vi "ABB Test report .vi"() -> (0 "error out":errorcluster)   [LabVIEW 2017]
uses:
  ABB global.vi
  <vilib>/Utility/NIReport.llb/NI_report.lvclass
panel:
  in  "Sign":bool
  out "Array":cluster{"String":string, "OK Button":bool}[](array[cluster])
  out "result string":string
  in  "Save":bool
  in  "View Pages":bool
  in  "Select page":u16(ring) items=["Cover Page", "Contents", "Pass/Fail Criteria", "Rated Data", " General Information", "Measurements", "No Load Test", "Short Circuit Test", "Heat Run", "Heat Run Data", "Cooling curve", "No Load Heat Run", "Heat Run Data", "No Load Cooling curve", "Bearing Run", "Bearing Run Data", "Efficiency", "Noise", "Noise Analysis 1", "Noise Analysis 2", "Bearing Inspection", "Instruments"]
  out "Message":string="Compiling Report...."
  in  "Select None":bool
  in  "Select All":bool
  out "Pages":string[](array[string])
  in  "Include":bool[](array[boolean])
  in  "Exit":bool
  in  "Print":bool
  in  "WebBrowser":refnum<k7>(container)
  # "Test Report"
  # "Include pages"
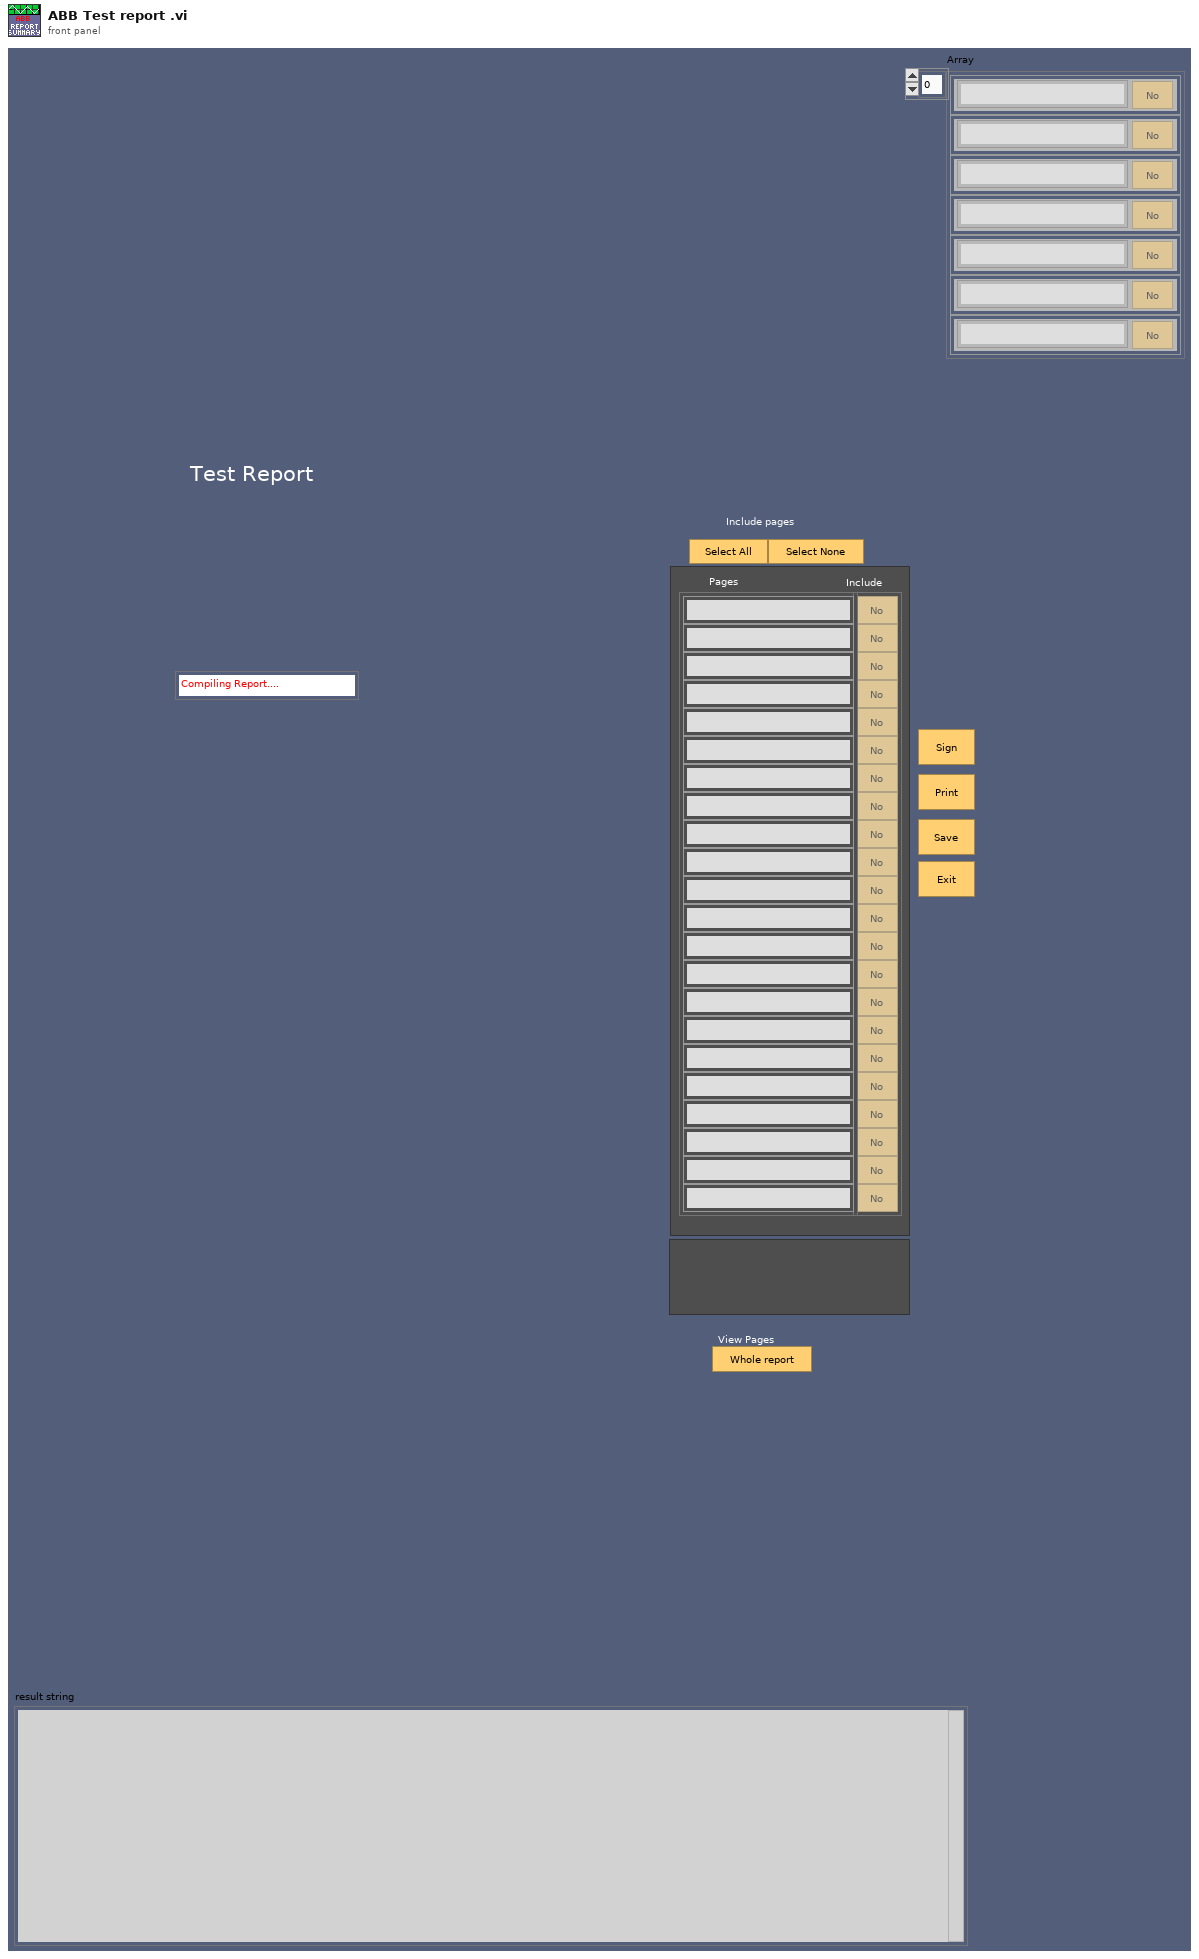
[diagram p1: front panel]
types:
  T1 = typedef "Generate Report Object Reference.ctl" = refnum<class "NI_report.lvclass">
  T2 = enum32{"existing file", "new file", "new or existing file", "existing dir", "new dir", "new or existing dir", "existing file (use LLBs)", "new file (use LLBs)", "new or existing file (use LLBs)", "new or existing file or directory (use LLBs)"}
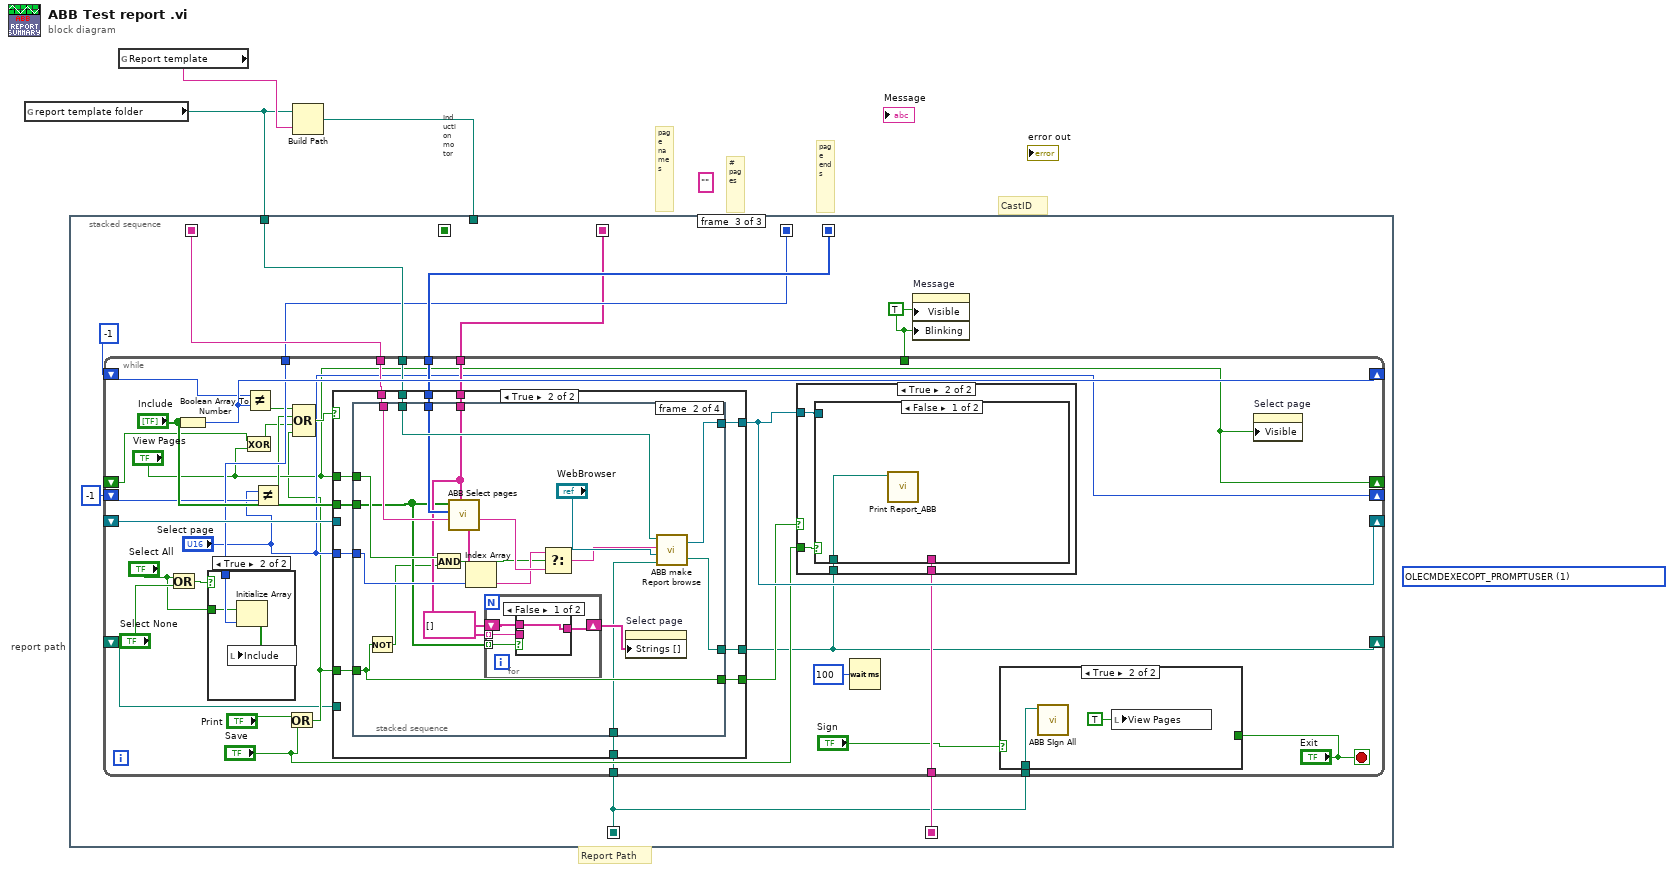
[diagram p0: block diagram]
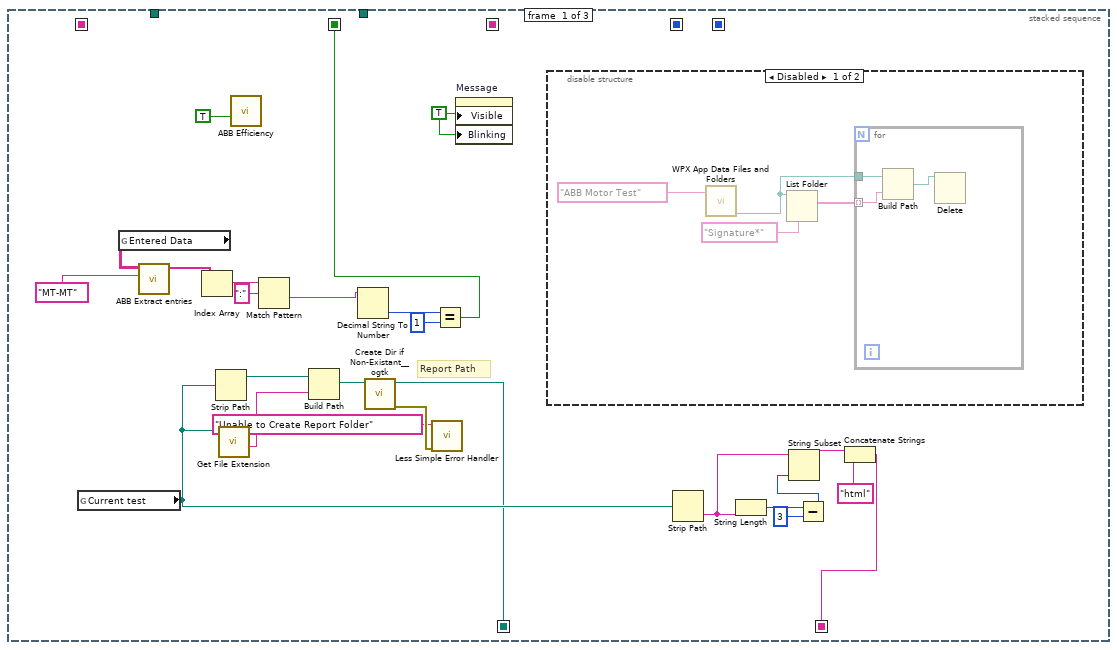
[diagram p2: hidden frame]
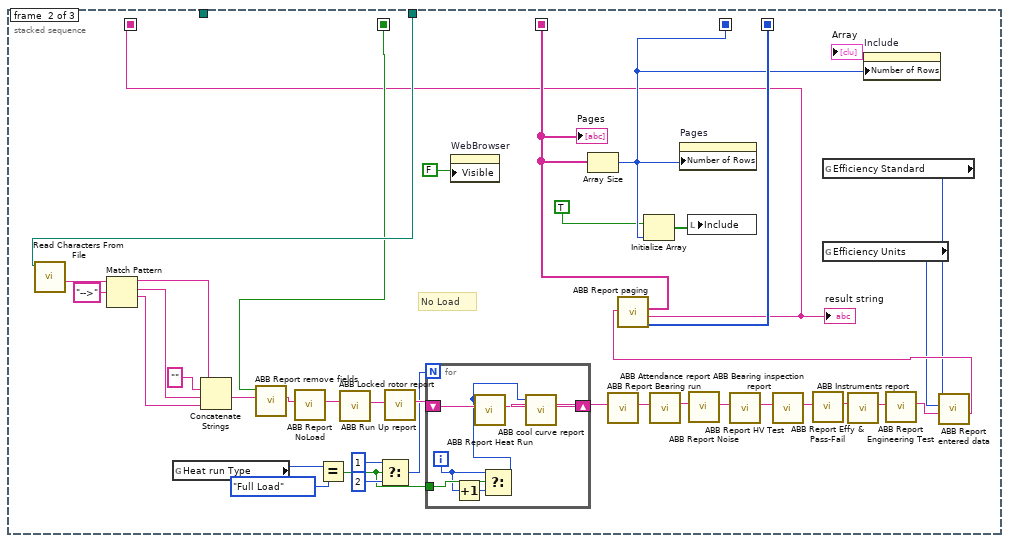
[diagram p4: hidden frame]
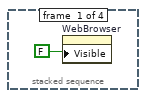
[diagram p8: hidden frame]
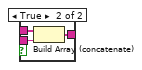
[diagram p9: hidden frame]
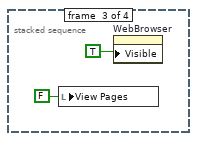
[diagram p10: hidden frame]
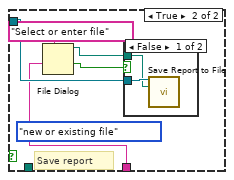
[diagram p13: hidden frame]
diagram:
  (unwired) 1 items=["OLECMDEXECOPT_DODEFAULT", "OLECMDEXECOPT_PROMPTUSER", "OLECMDEXECOPT_DONTPROMPTUSER", "OLECMDEXECOPT_SHOWHELP"] ("IE Print Options")
  (unwired) "" ("result string")
  # "Report Path"
  # "report path"
  # "Induction motor"
  # "page names"
  # "# pages"
  # "page ends"
  # "CastID"
  n1 = global read "ABB global.vi" "report template folder"() -> (w1:path)
  n2 = global read "ABB global.vi" "Report template"() -> (w2:string)
  n3 = Build Path(base path=w1, name or relative path=w2) -> (appended path=w3:path)
  n4 = stacked-sequence {
    seq-local: [_ w43 _] -> [_ _ w89]
    seq-local: [_ w65 _] -> [_ _ w87]
    seq-local: [_ w64 _] -> [_ _ w86]
    seq-local: [_ w60 _] -> [_ _ w85]
    seq-local: [w18 _ _] -> [_ w47 _]
    seq-local: [w11 _ _] -> [_ _ w82]
    seq-local: [w6 _ _] -> [_ _ w81]
    tunnel: w3 -> [_ w68 _]
    tunnel: w1 -> [_ _ w88]
    frame #0 {
      w28 = TRUE ("Visible")
      # "Report Path"
      n5 = global read "ABB global.vi" "Current test"() -> (w10:path)
      n6 = global read "ABB global.vi" "Entered Data"() -> (w26:string[][])
      n7 = call "ABB Extract entries.vi"("Entry ID"="MT-MT", "Entry table in"=w26) -> ("Selected Entries"=w24:string[])  [unwired: 9 in]
      n8 = Index Array(array=w24) -> (element=w23:string)  [unwired: 1 in]
      n9 = Strip Path(path=w10) -> (stripped path=w9:path)  [unwired: 1 out]
      n10 = call <vilib>:"Get File Extension.vi"("file"=w10) -> ("filename without extension"=w8:string)  [unwired: 6 in, 4 out]
      n11 = call "ABB Efficiency.vi"("auto save"=TRUE) -> ()  [unwired: 11 in]
      n12 = Match Pattern(string=w23, regular expression=":") -> (after substring=w21:string)  [unwired: 1 in, 3 out]
      n13 = Build Path(base path=w9, name or relative path=w8) -> (appended path=w7:path)
      n14 = Decimal String To Number(string=w21) -> (number=w20:i32)  [unwired: 2 in, 1 out]
      n15 = call <userlib>:"Create Dir if Non-Existant__ogtk.vi"("Directory Path"=w7) -> ("error out"=w5:errorcluster, "dup Directory Path"=w6:path)  [unwired: 8 in, 1 out]
      n16 = call "Less Simple Error Handler.vi"("message"="Unable to Create Report Folder", "error in"=w5) -> ()  [unwired: 4 in]
      n17 = Equal?(x=w20, y=1) -> (x = y?=w18:bool)
      n18 = property on="Message" class="Str"("Visible"=w28, "Blinking"=w28) -> ()  [unwired: 2 in, 2 out]
      n19 = disable-structure shown="Disabled" {
        frame Disabled {
          n20 = call "WPX App Data Files and Folders.vi"("ApplicationName"="ABB Motor Test") -> ("DataFolder"=w29:path)  [unwired: 7 in, 3 out]
          n21 = List Folder(path=w29, pattern="Signature*") -> (filenames=w30:string[])  [unwired: 2 in, 3 out]
          n22 = for {
            tunnel: w30 -> [w35] mode=indexing
            tunnel: w29 -> [w34]
            n23 = Build Path(base path=w34, name or relative path=w35) -> (appended path=w33:path)
            n24 = Delete(path (use dialog)=w33) -> ()  [unwired: 4 in, 3 out]
          }
        }
        frame Enabled {
        }
      }
      n25 = Strip Path(path=w10) -> (name=w15:string)  [unwired: 1 out]
      n26 = String Length(string=w15) -> (length=w17:i32)
      n27 = Subtract(x=w17, y=3) -> (x-y=w14:i32)
      n28 = String Subset(string=w15, length (rest)=w14) -> (substring=w13:string)  [unwired: 1 in]
      n29 = Concatenate Strings(w13, "html" ("string")) -> (w11:string)
    }
    frame #1 {
      # "No Load"
      n30 = call <vilib>:"Read Characters From File.vi"("file path (dialog if empty)"=w68) -> ("character string"=w73:string)  [unwired: 5 in, 3 out]
      n31 = Match Pattern(string=w73, regular expression="-->") -> (before substring=w71:string, match substring=w70:string, after substring=w69:string)  [unwired: 1 in, 1 out]
      n32 = global read "ABB global.vi" "Heat run Type"() -> (w55:enum16{"Full Load", "Partial- & No-Load"})
      n33 = Concatenate Strings(w71, "" ("string"), w70, w69) -> (w48:string)
      n34 = call "ABB Report remove fields.vi"("Report in"=w48, "Induction motor"=w47) -> ("Report out"=w39:string)  [unwired: 9 in]
      n35 = call "ABB Report NoLoad.vi"("Report in"=w39) -> ("Report out"=w58:string)  [unwired: 9 in, 1 out]
      n36 = Equal?(x=w55, y=enum16{"Full Load", "Partial Load"}."Full Load") -> (x = y?=w50:bool)
      n37 = call "ABB Locked rotor report.vi"("Report in"=w58) -> ("Report out"=w67:string)  [unwired: 9 in, 1 out]
      n38 = Select(t=1, s=w50, f=2) -> (s? t:f=w51:i32)
      n39 = call "ABB Run Up report.vi"("Report in"=w67) -> ("Report out"=w59:string)  [unwired: 10 in]
      n40 = for {
        N: w51 -> [_]
        shift-right: [w76] -> w40
        shift-left: w59 -> [w80]
        tunnel: w50 -> [w79]
        i -> [w78]
        n41 = Increment(x=w78) -> (x+1=w77:i32)
        n42 = Select(t=w78, s=w79, f=w77) -> (s? t:f=w74:i32)
        n43 = call "ABB Report Heat Run.vi"("Report in"=w80, "Heat run #"=w74) -> ("Report out"=w75:string)  [unwired: 9 in]
        n44 = call "ABB cool curve report.vi"("Report in"=w75, "Heat run #"=w74) -> ("Report out"=w76:string)  [unwired: 9 in]
      }
      n45 = property on="WebBrowser" class="AXCont"("Visible"=FALSE) -> ()  [unwired: 2 in, 2 out]
      n46 = call "ABB Report Bearing run.vi"("Report in"=w40) -> ("Report out"=w61:string)  [unwired: 10 in]
      n47 = call "ABB Attendance report.vi"("Report in"=w61) -> ("Report out"=w49:string)  [unwired: 10 in]
      n48 = call "ABB Report Noise.vi"("Report in"=w49) -> ("Report out"=w57:string)  [unwired: 10 in]
      n49 = call "ABB Report HV Test.vi"("Report in"=w57) -> ("Report out"=w45:string)  [unwired: 10 in]
      n50 = call "ABB Bearing inspection report.vi"("Report in"=w45) -> ("Report out"=w38:string)  [unwired: 10 in]
      n51 = call "ABB Report Effy & Pass-Fail.vi"("Report in"=w38) -> ("Report out"=w44:string)  [unwired: 10 in]
      n52 = global read "ABB global.vi" "Efficiency Standard"() -> (w37:u16)
      n53 = global read "ABB global.vi" "Efficiency Units"() -> (w36:u16)
      n54 = call "ABB Instruments report.vi"("Report in"=w44) -> ("Report out"=w42:string)  [unwired: 10 in]
      n55 = call "ABB Report Engineering Test.vi"("Report in"=w42) -> ("Report out"=w41:string)  [unwired: 10 in]
      n56 = call "ABB Report entered data.vi"("result string in"=w41, "Efficiency Units"=w36, "Efficiency Standard"=w37) -> ("result string out"=w46:string)  [unwired: 8 in]
      n57 = call "ABB Report paging.vi"("String"=w46) -> ("page ends"=w65:i32[], "result string"=w43:string, "Page Names"=w60:string[])  [unwired: 7 in, 1 out]
      "result string" <- w43
      "Pages" <- w60
      n58 = Array Size(array=w60) -> (size(s)=w64:i32)
      n59 = Initialize Array(TRUE, w64) -> (w63:bool[])
      n60 = property on="Pages" class="Arr (strict)"("Number of Rows"=w64) -> ()  [unwired: 2 in, 2 out]
      n61 = local write "Include"(w63) -> ()
      n62 = property on="Include" class="Arr (strict)"("Number of Rows"=w64) -> ()  [unwired: 2 in, 2 out]
    }
    frame #2 {
      w84 = TRUE ("Visible")
      n63 = while {
        shift-right: [w123] -> _
        shift-left: -1 -> [w122]
        tunnel: w89 -> [w120]
        tunnel: w88 -> [w121]
        shift-right: [w119] -> _
        shift-left: _ -> [w118]
        tunnel: w87 -> [w116]
        tunnel: w86 -> [w113]
        tunnel: w85 -> [w110]
        tunnel: w84 -> [_]
        shift-right: ["Select page"] -> _
        shift-left: -1 ("index") -> [w107]
        shift-right: ["View Pages"] -> _
        shift-left: _ -> [w104]
        tunnel: w82 -> [w97]
        shift-right: [w95] -> _
        shift-left: _ -> [w96]
        tunnel: w81 -> [w92]
        tunnel: w81 -> [w91]
        stop <- "Exit" stop-if-true
        n64 = Or(x="Select All", y="Select None") -> (x .or. y?=w111:bool)
        n65 = Boolean Array To Number(Boolean array="Include") -> (number=w123:u32)
        n66 = case shown="True" w111 {
          tunnel: w113 -> [_ w128]
          tunnel: "Select All" -> [_ w127]
          frame False {
          }
          frame True {
            n67 = Initialize Array(w127, w128) -> (w126:bool[])
            n68 = local write "Include"(w126) -> ()
          }
        }
        n69 = Exclusive Or(1:"View Pages", 2:w104) -> (0:w103:bool)
        n70 = Not Equal?(x=w122, y=w123) -> (x != y?=w108:bool)
        n71 = Not Equal?(x="Select page", y=w107) -> (x != y?=w106:bool)
        n72 = Or(x="Print", y="Save") -> (x .or. y?=w100:bool)
        n73 = Compound Arithmetic op=OR(w108, w106, w103, w100) -> (w109:bool)
        n74 = case shown="True" w109 {
          tunnel: w121 -> [_ w143]
          tunnel: w120 -> [_ w141]
          tunnel: [w131 w142] -> w119
          tunnel: w118 -> [w131 _]
          tunnel: "Include" -> [_ w140]
          tunnel: w116 -> [_ w139]
          tunnel: w110 -> [_ w138]
          tunnel: "View Pages" -> [_ w137]
          tunnel: "Select page" -> [_ w136]
          tunnel: w100 -> [w130 w135]
          tunnel: [w130 w134] -> w101
          tunnel: [w129 w133] -> w95
          tunnel: w96 -> [w129 _]
          tunnel: w91 -> [_ w132]
          frame False {
          }
          frame True {
            n75 = stacked-sequence {
              tunnel: w143 -> [_ w163 _ _]
              tunnel: [_ w162 _ _] -> w142
              tunnel: w141 -> [_ w161 _ _]
              tunnel: w140 -> [_ w152 _ _]
              tunnel: w139 -> [_ w160 _ _]
              tunnel: w138 -> [_ w153 _ _]
              tunnel: w137 -> [_ w155 _ _]
              tunnel: w136 -> [_ w154 _ _]
              tunnel: w135 -> [_ w147 _ _]
              tunnel: [_ w147 _ _] -> w134
              tunnel: [_ w146 _ _] -> w133
              tunnel: w132 -> [_ w145 _ _]
              frame #0 {
                n76 = property on="WebBrowser" class="AXCont"("Visible"=FALSE) -> ()  [unwired: 2 in, 2 out]
              }
              frame #1 {
                n77 = Not(x=w147) -> (.not. x?=w148:bool)
                n78 = And(x=w155, y=w148) -> (x .and. y?=w149:bool)
                n79 = call "ABB Select pages.vi"("Page Names"=w153, "Report in"=w161, "Page ends"=w160, "Page select"=w152) -> ("Report out"=w159:string, "Pages out"=w157:string[])  [unwired: 5 in, 1 out]
                n80 = Index Array(array=w157, index=w154) -> (element=w156:string)
                n81 = for {
                  tunnel: w153 -> [w167] mode=indexing
                  tunnel: w152 -> [w168] mode=indexing
                  shift-right: [w165] -> w150
                  shift-left: string[] [] -> [w166]
                  n82 = case shown="False" w168 {
                    tunnel: w167 -> [_ w172]
                    tunnel: w166 -> [w169 w171]
                    tunnel: [w169 w170] -> w165
                    frame False {
                    }
                    frame True {
                      n83 = Build Array (concatenate)(w171, w172) -> (w170:string[])
                    }
                  }
                }
                n84 = Select(t=w156, s=w149, f=w159) -> (s? t:f=w158:string)
                n85 = property on="Select page" class="Ring (strict)"("Strings []"=w150) -> ()  [unwired: 2 in, 2 out]
                n86 = call "ABB make Report browse.vi"("Report path"=w145, "WebBrowser"="WebBrowser", "result string"=w158, "report template folder"=w163) -> ("Report  path"=w146:path, "report out"=w162:T1)
              }
              frame #2 {
                n87 = local write "View Pages"(FALSE ("View Pages")) -> ()
                n88 = property on="WebBrowser" class="AXCont"("Visible"=TRUE) -> ()  [unwired: 2 in, 2 out]
              }
              frame #3 {
              }
            }
          }
        }
        n89 = case shown="True" w101 {
          tunnel: w119 -> [_ w178]
          tunnel: "Save" -> [_ w177]
          tunnel: w97 -> [_ w176]
          tunnel: w95 -> [_ w175]
          frame False {
          }
          frame True {
            n90 = case shown="False" w177 {
              tunnel: w178 -> [_ w184]
              tunnel: w176 -> [_ w183]
              tunnel: w175 -> [w179 _]
              frame False {
                n91 = call "Print Report_ABB.vi"("Report  path"=w179) -> ()  [unwired: 11 in]
              }
              frame True {
                (unwired) T2."new or existing file" ("select mode (2)")
                # "Save report"
                n92 = File Dialog(7:"Select or enter file" ("prompt"), 9:w183) -> (1:w180:bool, 3:w181:path)  [unwired: 5 in, 2 out]
                n93 = case shown="False" w180 {
                  tunnel: w184 -> [w186 _]
                  tunnel: w181 -> [w185 _]
                  frame False {
                    n94 = call-dynamic "Save Report to File.vi"("report in"=w186, "report file path"=w185) -> ()  [unwired: 12 in, 2 out]
                  }
                  frame True {
                  }
                }
              }
            }
          }
        }
        n95 = Wait (ms)(milliseconds to wait=u32 100) -> ()  [unwired: 1 out]
        n96 = case shown="True" "Sign" {
          tunnel: "Exit" -> [_ _]
          tunnel: w92 -> [_ w124]
          frame False {
          }
          frame True {
            n97 = call "ABB SIgn All.vi"("ImageFolder"=w124) -> ()  [unwired: 11 in]
            n98 = local write "View Pages"(TRUE ("View Pages")) -> ()
          }
        }
        n99 = property on="Select page" class="Ring (strict)"("Visible"="View Pages") -> ()  [unwired: 2 in, 2 out]
      }
      n100 = property on="Message" class="Str"("Visible"=w84, "Blinking"=w84) -> ()  [unwired: 2 in, 2 out]
    }
  }
